vi "Generate.vi"(8 "error in (no error)":errorcluster, 11 "Tirangle in":refnum<class "Tirangle.lvclass">) -> (0 "error out":errorcluster, 3 "Tirangle out":refnum<class "Tirangle.lvclass">)   [LabVIEW 2020, in "Tirangle.lvclass"]
uses:
  Tirangle.lvclass
  C:/Users/fflores/Documents/GitHub Projects/OOP-Concepts-in-LabVIEW/Design Patterns/Composite Pattern/Analog Waveform/Analog Waveform.lvclass
  Analog Waveform/Analog Waveform.lvclass/Analog Waveform.ctl
  Analog Waveform/Read Offset.vi
  Analog Waveform/Read Frequency.vi
  Analog Waveform/Read Amplitude.vi
  Analog Waveform/Read Phase.vi
  Analog Waveform/Write Waveform Data.vi
  <vilib>/measure/NI_MABase.lvlib
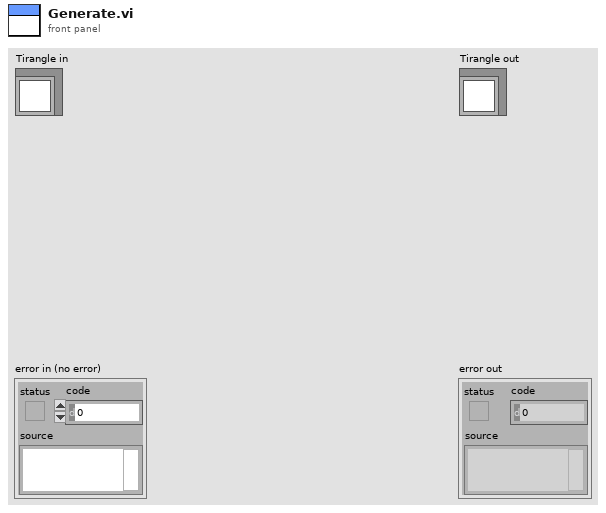
[diagram p1: front panel]
types:
  T1 = enum16{"Sine Wave", "Triangle Wave", "Square Wave", "Sawtooth Wave"}
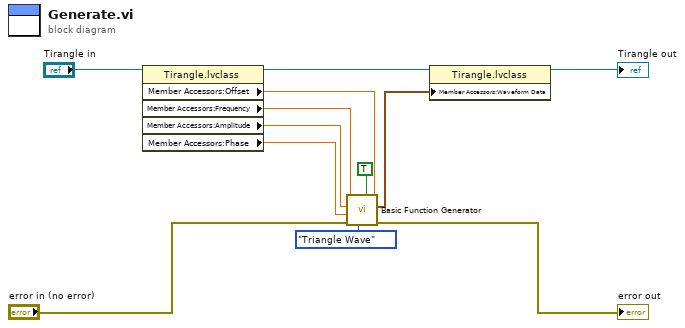
[diagram p0: block diagram]
diagram:
  n1 = property class="Tirangle.lvclass"(reference="Tirangle in") -> (reference out=w12:refnum<class "Tirangle.lvclass">, "Member Accessors:Offset"=w11:dbl, "Member Accessors:Frequency"=w10:dbl, "Member Accessors:Amplitude"=w9:dbl, "Member Accessors:Phase"=w8:dbl)  [unwired: 1 in, 1 out]
  n2 = call <vilib>:"Basic Function Generator.vi"("offset"=w11, "reset signal"=TRUE, "signal type"=T1."Triangle Wave", "error in (no error)"="error in (no error)", "phase"=w8, "amplitude"=w9, "frequency"=w10) -> ("error out"=→"error out":errorcluster, "signal out"=w6:waveform(dbl))  [unwired: 2 in, 1 out]
  n3 = property class="Tirangle.lvclass"(reference=w12, "Member Accessors:Waveform Data"=w6) -> (reference out=→"Tirangle out":refnum<class "Tirangle.lvclass">)  [unwired: 1 in, 1 out]
